vi "Read FilePath.vi"(8 "error in (no error)":errorcluster, 11 "GenericFileClass in":refnum<class "GenericFileClass.lvclass">) -> (0 "error out":errorcluster, 2 "FilePath":path=path "C:/TrigBoxSettings/Settings.ini", 3 "GenericFileClass out":refnum<class "GenericFileClass.lvclass">)   [LabVIEW 2013, in "GenericFileClass.lvclass"]
uses:
  GenericFileClass.lvclass
  GenericFileClass.lvclass/GenericFileClass.ctl
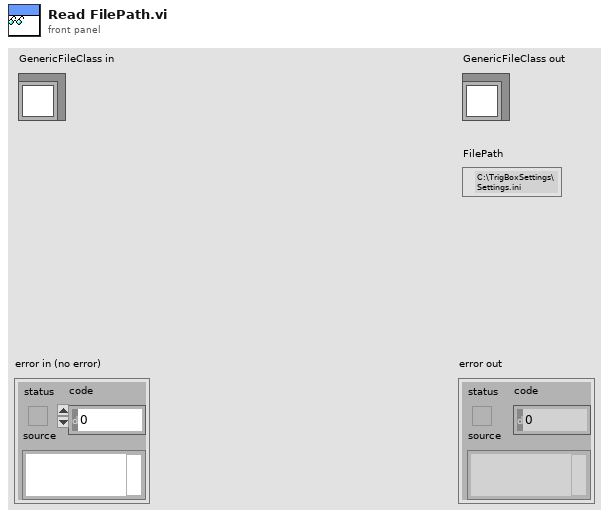
[diagram p1: front panel]
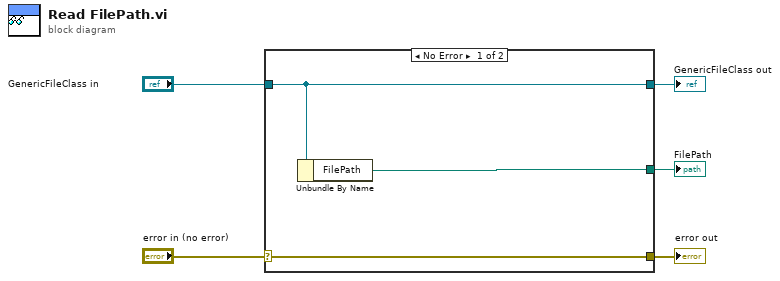
[diagram p0: block diagram]
diagram:
  n1 = case shown="No Error" "error in (no error)" {
    selector: "error in (no error)" -> [w8 w9]
    tunnel: [w8 w9] -> w4
    tunnel: [w7 w10] -> w2
    tunnel: "GenericFileClass in" -> [w7 w10]
    tunnel: [w6 _] -> w1
    frame No Error {
      n2 = Unbundle By Name(w7) -> ("FilePath"=w6:path)
    }
    frame Error {
    }
  }
  "error out" <- w4
  "GenericFileClass out" <- w2
  "FilePath" <- w1
